vi "Drive_with_Gyro.vi"(6 "Synchronication":enum16{"Start", "Wait"}(ring)=enum."Wait", 7 "Description":string, 8 "Command Info In":T1, 9 "Dis":dbl, 10 "Left":dbl, 11 "Right":dbl) -> (0 "Command Info Out":T1)   [LabVIEW 2015]
doc: "This VI notifies the subsystem to perform this command for the given duration, then go back to the default state. Synchronization determines whether this VI Starts the operation and returns immediately, or waits for the operation to complete. The first option is commonly used for TeleOp, and the second for Autonomous sequencing."
uses:
  <vilib>/Rock Robotics/WPI/Framework/Command Status Info.ctl
  <vilib>/Rock Robotics/WPI/Framework/Completion Status.ctl
  <vilib>/Rock Robotics/WPI/Framework/Completion Notifier.ctl
  Implementation/Drive Setpoints.ctl
  Implementation/Drive Operations.ctl
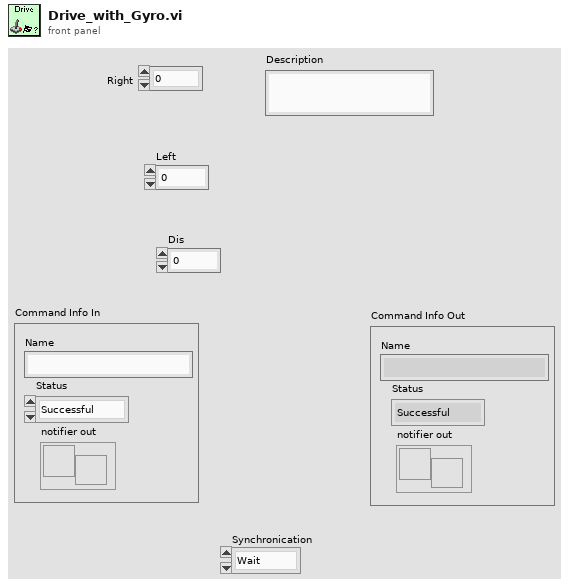
[diagram p1: front panel]
types:
  T1 = typedef "Command Status Info.ctl" = cluster{"Name":string, "Status":T2, "notifier out":T3}
  T2 = typedef "Completion Status.ctl" = enum16{"Successful", "Aborted", "Incomplete"}
  T3 = typedef "Completion Notifier.ctl" = refnum<notifier>
  T4 = typedef "Drive Setpoints.ctl" = cluster{"Operation":T5, "Left Setpoint":dbl, "Right Setpoint":dbl, "Duration":dbl, "Distance":dbl}
  T5 = typedef "Drive Operations.ctl" = enum16{"Reserve", "Read Current", "Immediate", "Drive for Time", "Drive for Distance", "Drive With Gyro"}
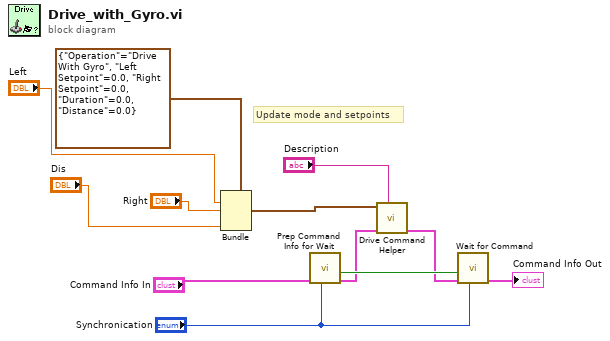
[diagram p0: block diagram]
diagram:
  # "Update mode and setpoints"
  n1 = Bundle(cluster=T4 {"Operation"=enum."Drive With Gyro", "Left Setpoint"=0.0, "Right Setpoint"=0.0, "Duration"=0.0, "Distance"=0.0} ("SubSystem Data"), "Left Setpoint"="Left", "Right Setpoint"="Right", "Distance"="Dis") -> (w5:T4)  [unwired: 2 in]
  n2 = call <vilib>:"Prep Command Info for Wait.vi"("Synchronication"="Synchronication", "Command Info"="Command Info In") -> ("Command Info"=w9:T1, "Allocated"=w10:bool)  [unwired: 8 in]
  n3 = call "Drive Command Helper.vi"("Description"="Description", "Command Info In"=w9, "SubSystem Data"=w5) -> ("Command Info Out"=w6:T1)  [unwired: 7 in, 1 out]
  n4 = call <vilib>:"Wait for Command.vi"("Synchronication"="Synchronication", "Command Info in"=w6, "Allocated"=w10) -> ("Command Info out"=→"Command Info Out":T1)  [unwired: 8 in]
